vi "测试读设置.vi"() -> ()   [LabVIEW 2012, in "m_Lib.lvlib"]
uses:
  <userlib>/m_Lib/Setting/Demo/Data.ctl
  <userlib>/m_Lib/m_Lib.lvlib
panel:
  out "Error_Out":errorcluster
  out "簇":T1
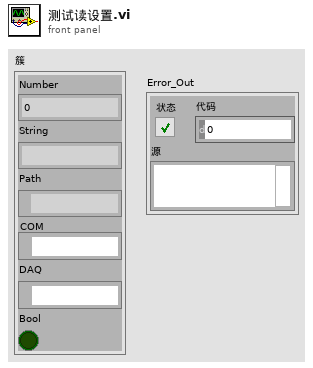
[diagram p1: front panel]
types:
  T1 = typedef "m_Lib.lvlib/Data.ctl" = cluster{"Number":u32, "String":string, "Path":path, "COM":refnum<visa-resource-name>, "DAQ":tag, "Bool":bool}
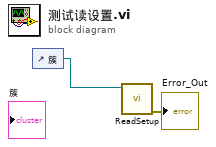
[diagram p0: block diagram]
diagram:
  n1 = control-ref of="簇"() -> (w2:refnum<vi>)
  n2 = call <userlib>:"ReadSetup.vi"("Cluster_Quotes"=w2) -> ("Error_Out"=→"Error_Out":errorcluster)  [unwired: 10 in]
